vi "25mean (delete).vi"(0 "input data":dbl, 1 "reset":bool) -> (4 "mean":dbl, 10 "output valid":bool)   [LabVIEW 2019]
doc: "Calculates the mean, variance, and/or standard deviation of an input signal. This Express VI analyzes discrete frames of data rather than analyzing data continuously. This Express VI waits for N cycles to collect a frame of data before returning one valid output, where N is the number of samples in each frame. It then waits for another N cycles to return another valid output.\n--------------------\n\nThis Express VI is configured as follows:\n\n<b>Number of samples</b>\n25\n\n<b>Statistics</b>\nmean\n\n<b>Execution Mode</b>\nOutside single-cycle Timed Loop"
uses:
  <vilib>/Platform/TimedLoop/XDataNode/wakeup.ctl
  <vilib>/Platform/TimedLoop/XDataNode/XDNodeRunTimeDep.lvlib
  <vilib>/Platform/TimedLoop/XDataNode/nitl_modes.ctl
  <vilib>/Platform/TimedLoop/XDataNode/timing_clust.ctl
  <vilib>/Platform/TimedLoop/XDataNode/XDataNode.xnode
  <vilib>/rvi/FXPMathLib/basic elements/FxpIntAccumulator/XNode/nifxpmath_IntAccumulator.xnode
  <vilib>/rvi/FXPMathLib/FxpMul/XNode/nifxpmath_Multiplier.xnode
  <vilib>/rvi/FXPMathLib/basic elements/FxpIntAccumulator/simVIs/DllFxpIntAccumulator_sub.vi
  <vilib>/rvi/FXPMathLib/basic elements/FxpIntAccumulator/subVIs/nifxpmath_IntAccumulator_SimConfig.ctl
  <vilib>/rvi/FXPMathLib/sim/FxpSim.dll
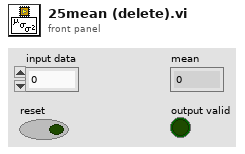
[diagram p1: front panel]
types:
  T1 = typedef "XDNodeRunTimeDep.lvlib/timing_clust.ctl" = cluster{"Expected End [f-1]":u64, "Actual End [f-1]":u64, "Finished Late? [f-1]":bool, "Expected End [i-1]":u64, "Actual End [i-1]":u64, "Finished Late? [i-1]":bool, "Expected Start [i]":u64, "Actual Start [i]":u64, "Expected Start [f]":u64, "Actual Start [f]":u64, "Source Name":string, "Structure Name":string, "Period":i64, "Deadline":i64, "Offset":i64, "Start":i64, "Priority":i32, "Timeout":i32, "Mode":T2, "Wakeup Reason":T3, "Error":errorcluster, "Source Type":string, "Secondary Source Type":string, "Global End Time":u64, "Global Start Time":u64, "Frame Duration":u64, "Iteration Duration":u64, "Assigned CPU":i32, "I/O Scan Engine Mode":u32}
  T2 = typedef "XDNodeRunTimeDep.lvlib/nitl_modes.ctl" = enum32{"No Change", "Process missed periods, maintain original phase", "Discard missed periods, maintain original phase", "Process missed periods, ignore original phase", "Discard missed periods, ignore original phase"}
  T3 = typedef "XDNodeRunTimeDep.lvlib/wakeup.ctl" = enum32{"Normal", "Aborted", "Asynchronous wakeup", "Timing source error", "Timed loop error", "Timeout"}
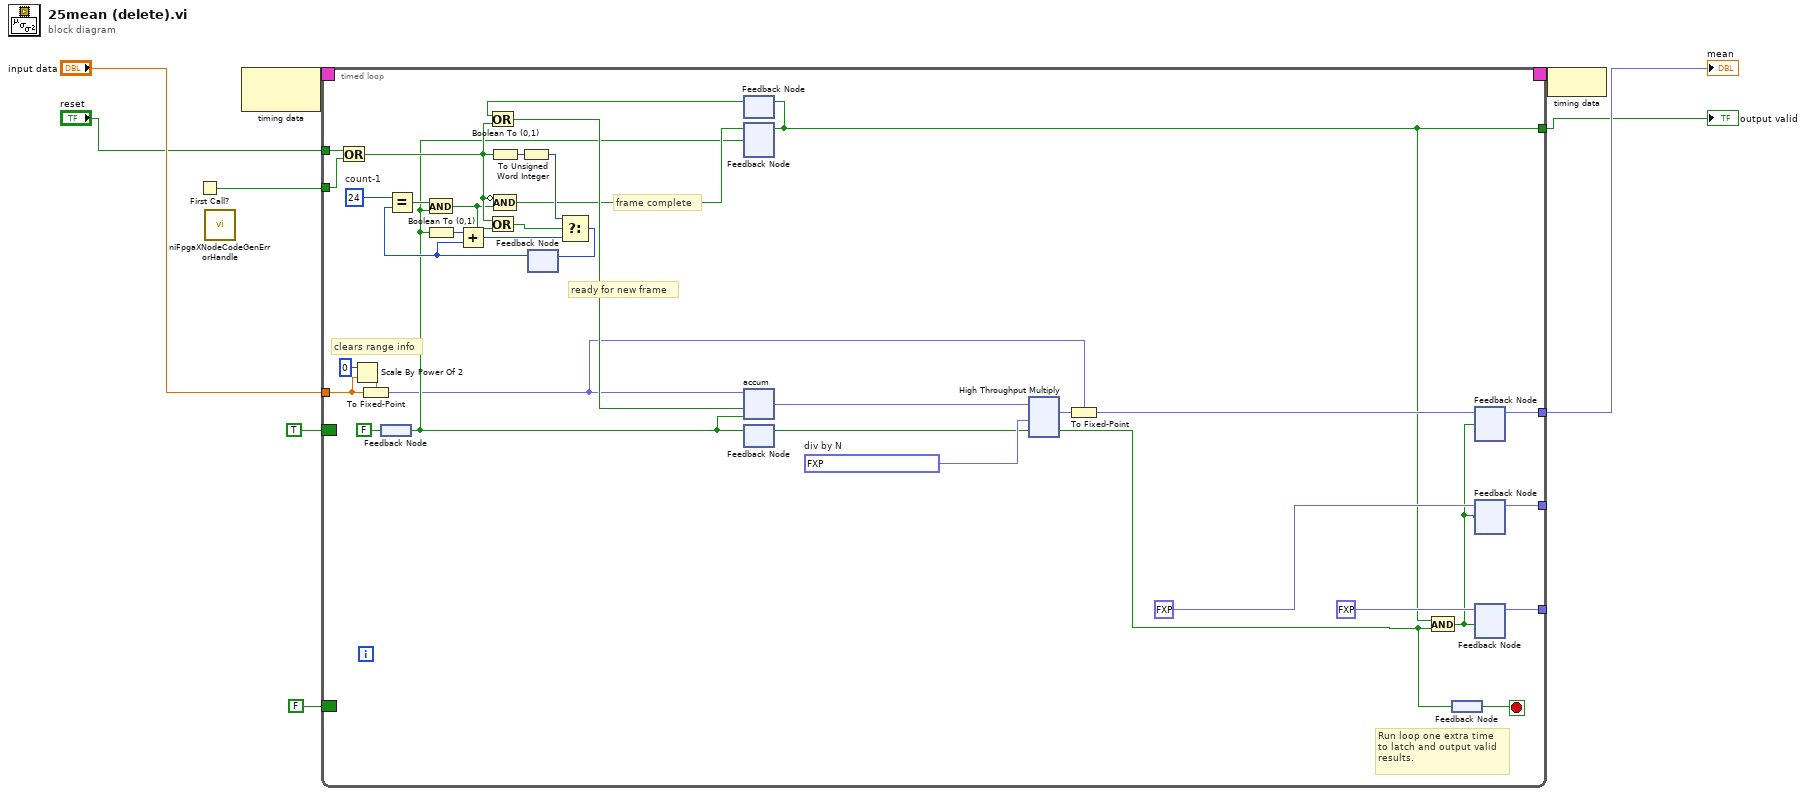
[diagram p0: block diagram]
diagram:
  n1 = First Call?() -> (First Call?: T/F=w1:bool)
  n2 = call <vilib>:"niFpgaXNodeCodeGenErrorHandle.vi"() -> ()  [unwired: 1 in]
  n3 = node-c288() -> (w5:T1)  [unwired: 1 in]
  n4 = timed-loop {
    tunnel: [w20] -> w7
    tunnel: "input data" -> [w12]
    tunnel: "reset" -> [w41]
    tunnel: w1 -> [w40]
    tunnel: [w18] -> _
    tunnel: [w16] -> _
    tunnel: [w15] -> w6
    timing: w5 -> [_]
    timing-out: [_] -> w4
    border: TRUE -> [_]
    border: FALSE ("output valid") -> [_]
    stop <- w13 stop-if-true
    w31 = fxp<+,17,-4> 0.039999961853027344  # div by N
    w45 = u16 24  # count-1
    # "Run loop one extra time\nto latch and output valid\nresults."
    # "clears range info"
    # "frame complete"
    # "ready for new frame"
    n5 = Or(x=w41, y=w40) -> (x .or. y?=w35:bool)
    n6 = Scale By Power Of 2(n=0, x=w12) -> (x*2^n=w24:dbl)
    n7 = To Fixed-Point(fixed-point type=w24, number=w12) -> (fixed-point=w11:fxp<+/-,21,-4>)
    n8 = feedback #1() -> (w22:bool)
    n9 = feedback-in #1(FALSE) -> ()
    n10 = Boolean To (0,1)(Boolean=w22) -> (0, 1=w39:i16)
    n11 = Boolean To (0,1)(Boolean=w35) -> (0, 1=w44:i16)
    n12 = To Unsigned Word Integer(number=w44) -> (unsigned 16bit integer=w43:u16)
    n13 = feedback #2() -> (w32:u16)  [unwired: 1 in]
    n14 = Equal?(x=w45, y=w32) -> (x = y?=w37:bool)
    n15 = And(x=w37, y=w22) -> (x .and. y?=w34:bool)
    n16 = Add(x=w39, y=w32) -> (x+y=w38:u16)
    n17 = Or(x=w35, y=w34) -> (x .or. y?=w36:bool)
    n18 = Compound Arithmetic op=AND(invert w35, w34) -> (w28:bool)
    n19 = Select(t=w43, s=w36, f=w38) -> (s? t:f=w42:u16)
    n20 = feedback-in #2(w42) -> ()
    n21 = feedback #3() -> (w33:bool)  [unwired: 1 in]
    n22 = Or(x=w33, y=w35) -> (x .or. y?=w29:bool)
    n23 = feedback-in #4(w28, w22) -> ()
    n24 = feedback #4() -> (w15:bool)  [unwired: 1 in]
    n25 = feedback-in #3(w15) -> ()
    n26 = xnode "accum"("x"=w11, "load (F)"=w29, "enable (T)"=w22) -> ("s"=w30:fxp<+/-,26,1>)  [unwired: 2 in, 1 out]
    n27 = feedback-in #5(w22) -> ()
    n28 = feedback #5() -> (w27:bool)  [unwired: 1 in]
    n29 = xnode ("High Throughput Multiply")("x"=w30, "y"=w31, "input valid"=w27) -> ("x*y"=w10:fxp<+/-,43,-3>, "output valid"=w26:bool)  [unwired: 1 in, 1 out]
    n30 = To Fixed-Point(fixed-point type=w11, number=w10) -> (fixed-point=w21:fxp<+/-,21,-4>)
    n31 = And(x=w15, y=w26) -> (x .and. y?=w14:bool)
    n32 = feedback-in #6(w26) -> ()
    n33 = feedback #6() -> (w13:bool)
    n34 = feedback #7() -> (w20:fxp<+/-,21,-4>)  [unwired: 1 in]
    n35 = feedback-in #7(w21, w14) -> ()
    n36 = feedback #8() -> (w18:fxp<+,63,1>)  [unwired: 1 in]
    n37 = feedback-in #8(fxp<+,63,1> 0.0 ("square type"), w14) -> ()
    n38 = feedback #9() -> (w16:fxp<+,32,1>)  [unwired: 1 in]
    n39 = feedback-in #9(fxp<+,32,1> 0.0 ("square type"), w14) -> ()
  }
  "mean" <- w7
  "output valid" <- w6
  n40 = node-c288(w4) -> ()
